vi "Calculate Plot Range.vi"(8 "error in (no error)":errorcluster, 9 "Coordinates System":enum16{"Cartesian", "Cylindrical", "Spherical"}(ring), 10 "3D Ribbon Datatype.lvclass in":refnum<class "3D Ribbon Datatype.lvclass">, 11 "Plot Representation In":T1) -> (0 "error out":errorcluster, 2 "3D Ribbon Datatype.lvclass out":refnum<class "3D Ribbon Datatype.lvclass">, 3 "Plot Representation Out":T1)   [LabVIEW 2017, in "3D Ribbon Datatype.lvclass"]
uses:
  <vilib>/Math Plots/3D Math Plots/3D Ribbon/3D Ribbon Datatype/3D Ribbon Datatype.lvclass
  <vilib>/Math Plots/3D Math Plots/3D Plot/3D Plot/Typedef/Plot Representation.ctl
  <vilib>/Math Plots/3D Math Plots/3D Plot/3D Plot/Typedef/Range Clusters.ctl
  <vilib>/Math Plots/3D Math Plots/3D Plot/3D Plot/Typedef/Mesh Data.ctl
  <vilib>/Math Plots/3D Math Plots/3D Plot/3D Plot Datatype/3D Plot Datatype.lvclass
  <vilib>/Math Plots/3D Math Plots/3D Plot/3D Plot/3D Plot.lvclass
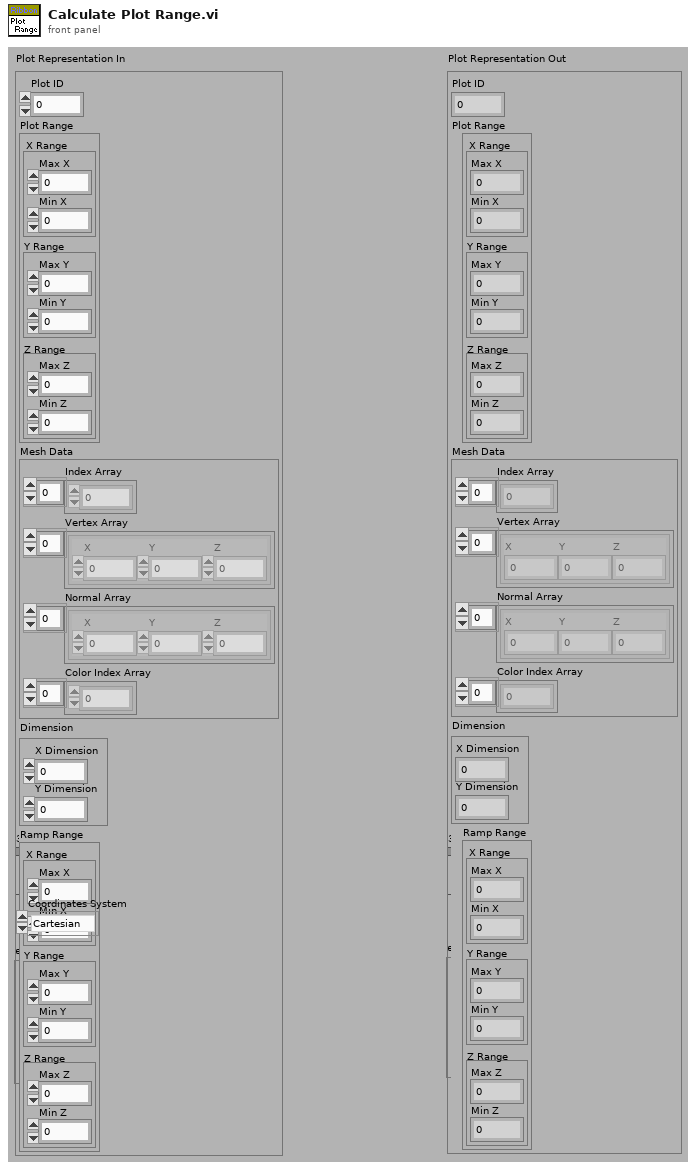
[diagram p1: front panel]
types:
  T1 = typedef "3D Plot.lvclass/Plot Representation.ctl" = cluster{"Plot ID":i32, "Plot Range":T2, "Mesh Data":T3, "Dimension":cluster{"X Dimension":i32, "Y Dimension":i32}, "Ramp Range":T2}
  T2 = typedef "3D Plot.lvclass/Range Clusters.ctl" = cluster{"X Range":cluster{"Max X":sgl, "Min X":sgl}, "Y Range":cluster{"Max Y":sgl, "Min Y":sgl}, "Z Range":cluster{"Max Z":sgl, "Min Z":sgl}}
  T3 = typedef "3D Plot.lvclass/Mesh Data.ctl" = cluster{"Index Array":u32[], "Vertex Array":cluster{"X":sgl, "Y":sgl, "Z":sgl}[], "Normal Array":cluster{"X":sgl, "Y":sgl, "Z":sgl}[], "Color Index Array":i32[]}
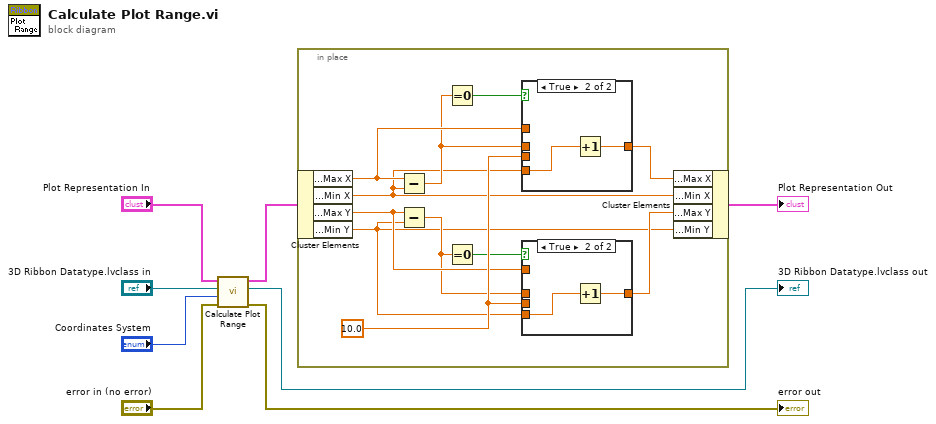
[diagram p0: block diagram]
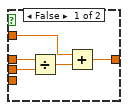
[diagram p2: hidden frame]
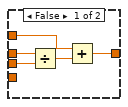
[diagram p3: hidden frame]
diagram:
  n1 = call-parent "Calculate Plot Range.vi"("error in (no error)"="error in (no error)", "Coordinates System"="Coordinates System", "3D Plot Datatype.lvclass in"="3D Ribbon Datatype.lvclass in", "Plot Representation In"="Plot Representation In") -> ("error out"=→"error out":errorcluster, "3D Plot Datatype.lvclass out"=→"3D Ribbon Datatype.lvclass out":refnum<class "3D Ribbon Datatype.lvclass">, "Plot Representation Out"=w1:T1)  [unwired: 5 out]
  n2 = in-place {
    w19 = sgl 10.0 ("y")
    n3 = in-place-cluster #1(w1) -> ("Plot Range.X Range.Max X"=w18:sgl, "Plot Range.X Range.Min X"=w12:sgl, "Plot Range.Y Range.Max Y"=w15:sgl, "Plot Range.Y Range.Min Y"=w9:sgl)
    n4 = Subtract(x=w18, y=w12) -> (x-y=w14:sgl)
    n5 = Subtract(x=w15, y=w9) -> (x-y=w10:sgl)
    n6 = Equal To 0?(x=w14) -> (x = 0?=w13:bool)
    n7 = Equal To 0?(x=w10) -> (x = 0?=w11:bool)
    n8 = case shown="True" w13 {
      tunnel: w19 -> [w31 _]
      tunnel: w18 -> [w29 _]
      tunnel: [w28 w32] -> w17
      tunnel: w14 -> [w27 _]
      tunnel: w12 -> [_ w33]
      frame False {
        n9 = Divide(x=w27, y=w31) -> (x/y=w30:sgl)
        n10 = Add(x=w29, y=w30) -> (x+y=w28:sgl)
      }
      frame True {
        n11 = Increment(x=w33) -> (x+1=w32:sgl)
      }
    }
    n12 = case shown="True" w11 {
      tunnel: w19 -> [w24 _]
      tunnel: [w22 w25] -> w16
      tunnel: w15 -> [w21 _]
      tunnel: w10 -> [w20 _]
      tunnel: w9 -> [_ w26]
      frame False {
        n13 = Divide(x=w20, y=w24) -> (x/y=w23:sgl)
        n14 = Add(x=w21, y=w23) -> (x+y=w22:sgl)
      }
      frame True {
        n15 = Increment(x=w26) -> (x+1=w25:sgl)
      }
    }
    n16 = in-place-cluster #1("Plot Range.X Range.Max X"=w17, "Plot Range.X Range.Min X"=w12, "Plot Range.Y Range.Max Y"=w16, "Plot Range.Y Range.Min Y"=w9) -> (→"Plot Representation Out":T1)
  }
